vi "methane_reactor_setup.vi"() -> (2 "spec_file":path)   [LabVIEW 2019]
uses:
  lib/libSimulationControl/libSimulationControl.lvlib
  lib/libCheckpointUpdate/libCheckpointUpdate.lvlib
panel:
  # "*******************************************************************\nBiogas Plant Control\n\nAuthor: Paul Zügel\nGCSC-Frankfurt am Main 2020\n\n*******************************************************************"
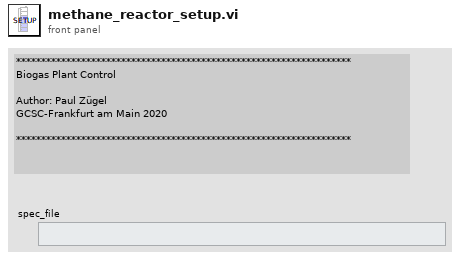
[diagram p1: front panel]
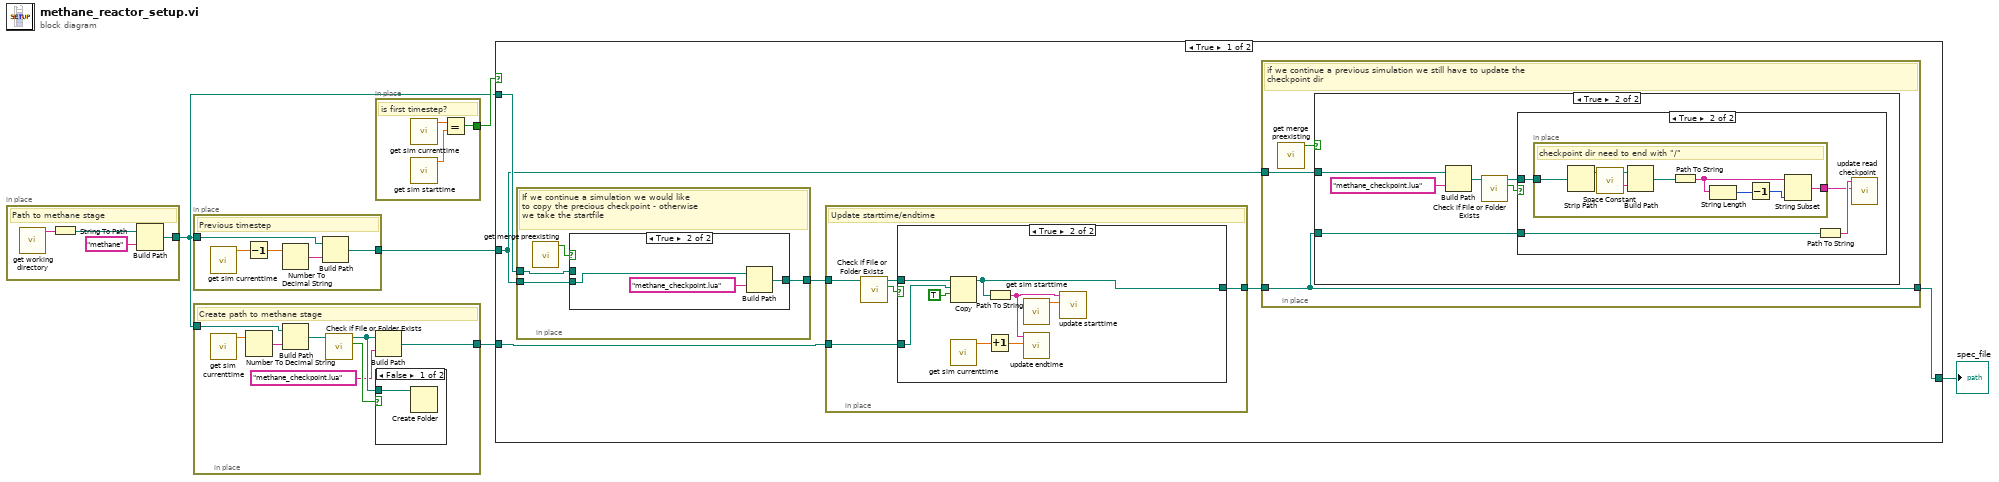
[diagram p0: block diagram]
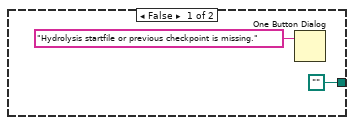
[diagram p3: hidden frame]
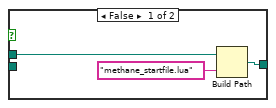
[diagram p4: hidden frame]
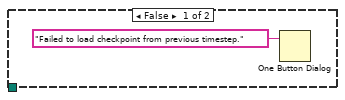
[diagram p6: hidden frame]
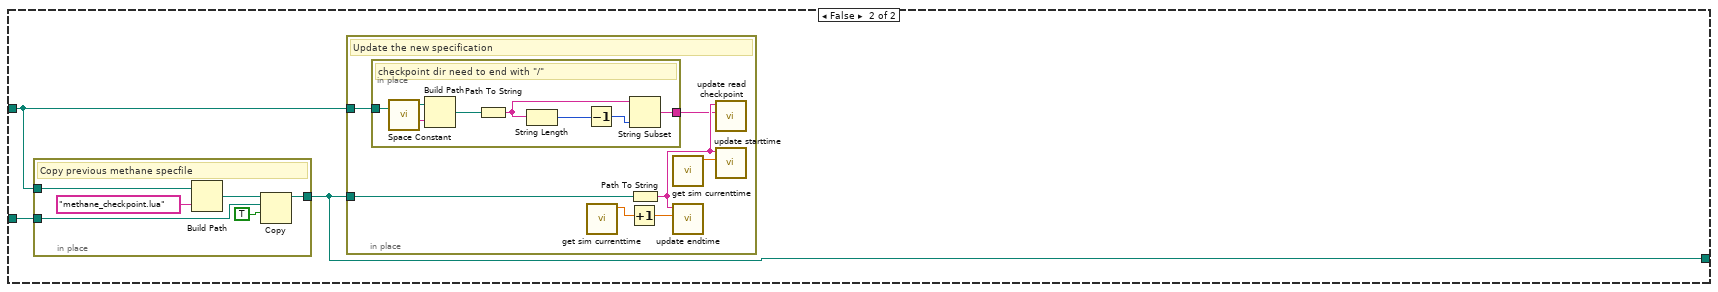
[diagram p7: hidden frame]
diagram:
  n1 = in-place {
    in-place-border: [w8] -> w1
    # "Path to methane stage"
    n2 = call "get working directory.vi"() -> ("function return"=w9:string)  [unwired: 10 in, 1 out]
    n3 = String To Path(string=w9) -> (path=w6:path)
    n4 = Build Path(base path=w6, name or relative path="methane" ("string")) -> (appended path=w8:path)
  }
  n5 = in-place {
    in-place-border: w1 -> [w13]
    in-place-border: [w11] -> w2
    # "Previous timestep"
    n6 = call "get sim currenttime.vi"() -> ("current_time"=w10:dbl)  [unwired: 10 in, 1 out]
    n7 = Decrement(x=w10) -> (x-1=w14:dbl)
    n8 = Number To Decimal String(number=w14) -> (decimal integer string=w12:string)  [unwired: 1 in]
    n9 = Build Path(base path=w13, name or relative path=w12) -> (appended path=w11:path)
  }
  n10 = in-place {
    in-place-border: [w17] -> w3
    in-place-border: w1 -> [w15]
    # "Create path to methane stage"
    n11 = call "get sim currenttime.vi"() -> ("current_time"=w16:dbl)  [unwired: 10 in, 1 out]
    n12 = Number To Decimal String(number=w16) -> (decimal integer string=w21:string)  [unwired: 1 in]
    n13 = Build Path(base path=w15, name or relative path=w21) -> (appended path=w20:path)
    n14 = call <vilib>:"Check if File or Folder Exists.vi"("path"=w20) -> ("file or folder exists?"=w22:bool, "dup path"=w19:path)  [unwired: 8 in, 1 out]
    n15 = Build Path(base path=w19, name or relative path="methane_checkpoint.lua" ("string")) -> (appended path=w17:path)
    n16 = case shown="False" w22 {
      tunnel: w19 -> [w23 _]
      frame False {
        n17 = Create Folder(path (use dialog)=w23) -> ()  [unwired: 2 in, 3 out]
      }
      frame True {
      }
    }
  }
  n18 = in-place {
    in-place-border: [w26] -> w5
    # "is first timestep?"
    n19 = call "get sim currenttime.vi"() -> ("current_time"=w24:dbl)  [unwired: 10 in, 1 out]
    n20 = call "get sim starttime.vi"() -> ("sim_starttime"=w25:dbl)  [unwired: 10 in, 1 out]
    n21 = Equal?(x=w24, y=w25) -> (x = y?=w26:bool)
  }
  n22 = case shown="True" w5 {
    tunnel: [w32 w81] -> w4
    tunnel: w3 -> [w28 w82]
    tunnel: w2 -> [w30 w80]
    tunnel: w1 -> [w31 _]
    frame True {
      n23 = in-place {
        in-place-border: [w51] -> w29
        in-place-border: w31 -> [w49]
        in-place-border: w30 -> [w48]
        # "If we continue a simulation we would like\nto copy the precious checkpoint - otherwise\nwe take the startfile"
        n24 = call "get merge preexisting.vi"() -> ("function return"=w50:bool)  [unwired: 10 in, 1 out]
        n25 = case shown="True" w50 {
          tunnel: [w53 w56] -> w51
          tunnel: w49 -> [w52 _]
          tunnel: w48 -> [_ w55]
          frame False {
            # "Copy base specification and update starttime/endtime"
            n26 = Build Path(base path=w52, name or relative path="methane_startfile.lua") -> (appended path=w53:path)
          }
          frame True {
            # "Copy previous hydrolysis spec file"
            n27 = Build Path(base path=w55, name or relative path="methane_checkpoint.lua" ("string")) -> (appended path=w56:path)
          }
        }
      }
      n28 = in-place {
        in-place-border: w29 -> [w35]
        in-place-border: w28 -> [w34]
        in-place-border: [w33] -> w27
        # "Update starttime/endtime"
        n29 = call <vilib>:"Check if File or Folder Exists.vi"("path"=w35) -> ("file or folder exists?"=w36:bool, "dup path"=w37:path)  [unwired: 8 in, 1 out]
        n30 = case shown="True" w36 {
          tunnel: [path "" w47] -> w33
          tunnel: w37 -> [_ w44]
          tunnel: w34 -> [_ w43]
          frame False {
            n31 = One Button Dialog(message="Hydrolysis startfile or previous checkpoint is missing.") -> ()  [unwired: 1 in, 1 out]
          }
          frame True {
            # "Update starttime/endtime"
            n32 = Copy(9:TRUE ("overwrite (F)"), 10:w43, 11:w44) -> (3:w47:path)  [unwired: 2 in, 2 out]
            n33 = call "get sim currenttime.vi"() -> ("current_time"=w42:dbl)  [unwired: 10 in, 1 out]
            n34 = Increment(x=w42) -> (x+1=w41:dbl)
            n35 = Path To String(path=w47) -> (string=w45:string)
            n36 = call "get sim starttime.vi"() -> ("sim_starttime"=w40:dbl)  [unwired: 10 in, 1 out]
            n37 = call "update endtime.vi"("endtime"=w41, "spec_dir"=w45) -> ()  [unwired: 9 in, 1 out]
            n38 = call "update starttime.vi"("starttime"=w40, "spec_dir"=w45) -> ()  [unwired: 9 in, 1 out]
          }
        }
      }
      n39 = in-place {
        in-place-border: w27 -> [w58]
        in-place-border: [w58] -> w32
        in-place-border: w30 -> [w59]
        # "if we continue a previous simulation we still have to update the \ncheckpoint dir"
        n40 = call "get merge preexisting.vi"() -> ("function return"=w60:bool)  [unwired: 10 in, 1 out]
        n41 = case shown="True" w60 {
          tunnel: w59 -> [_ w65]
          tunnel: w58 -> [_ w61]
          frame False {
          }
          frame True {
            n42 = Build Path(base path=w65, name or relative path="methane_checkpoint.lua" ("string")) -> (appended path=w64:path)
            n43 = call <vilib>:"Check if File or Folder Exists.vi"("path"=w64) -> ("file or folder exists?"=w62:bool, "dup path"=w63:path)  [unwired: 8 in, 1 out]
            n44 = case shown="True" w62 {
              tunnel: w63 -> [_ w69]
              tunnel: w61 -> [_ w70]
              frame False {
                n45 = One Button Dialog(message="Failed to load checkpoint from previous timestep.") -> ()  [unwired: 1 in, 1 out]
              }
              frame True {
                n46 = in-place {
                  in-place-border: w69 -> [w79]
                  in-place-border: [w72] -> w68
                  # "checkpoint dir need to end with \"/\""
                  n47 = Strip Path(path=w79) -> (stripped path=w73:path)  [unwired: 1 out]
                  n48 = call <vilib>:"Space Constant.vi"() -> ("String"=w74:string)
                  n49 = Build Path(base path=w73, name or relative path=w74) -> (appended path=w77:path)
                  n50 = Path To String(path=w77) -> (string=w78:string)
                  n51 = String Length(string=w78) -> (length=w76:i32)
                  n52 = Decrement(x=w76) -> (x-1=w75:i32)
                  n53 = String Subset(string=w78, length (rest)=w75) -> (substring=w72:string)  [unwired: 1 in]
                }
                n54 = Path To String(path=w70) -> (string=w71:string)
                n55 = call "update read checkpoint.vi"("checkpoint_dir"=w68, "spec_dir"=w71) -> ()  [unwired: 9 in, 1 out]
              }
            }
          }
        }
      }
    }
    frame False {
      n56 = in-place {
        in-place-border: w82 -> [w87]
        in-place-border: [w84] -> w81
        in-place-border: w80 -> [w83]
        # "Copy previous methane specfile"
        n57 = Build Path(base path=w83, name or relative path="methane_checkpoint.lua" ("string")) -> (appended path=w86:path)
        n58 = Copy(9:TRUE ("overwrite (F)"), 10:w87, 11:w86) -> (3:w84:path)  [unwired: 2 in, 2 out]
      }
      n59 = in-place {
        in-place-border: w81 -> [w95]
        in-place-border: w80 -> [w89]
        # "Update the new specification"
        n60 = in-place {
          in-place-border: [w97] -> w90
          in-place-border: w89 -> [w96]
          # "checkpoint dir need to end with \"/\""
          n61 = call <vilib>:"Space Constant.vi"() -> ("String"=w98:string)
          n62 = Build Path(base path=w96, name or relative path=w98) -> (appended path=w101:path)
          n63 = Path To String(path=w101) -> (string=w102:string)
          n64 = String Length(string=w102) -> (length=w100:i32)
          n65 = Decrement(x=w100) -> (x-1=w99:i32)
          n66 = String Subset(string=w102, length (rest)=w99) -> (substring=w97:string)  [unwired: 1 in]
        }
        n67 = call "get sim currenttime.vi"() -> ("current_time"=w92:dbl)  [unwired: 10 in, 1 out]
        n68 = Increment(x=w92) -> (x+1=w91:dbl)
        n69 = Path To String(path=w95) -> (string=w94:string)
        n70 = call "get sim currenttime.vi"() -> ("current_time"=w93:dbl)  [unwired: 10 in, 1 out]
        n71 = call "update endtime.vi"("endtime"=w91, "spec_dir"=w94) -> ()  [unwired: 9 in, 1 out]
        n72 = call "update read checkpoint.vi"("checkpoint_dir"=w90, "spec_dir"=w94) -> ()  [unwired: 9 in, 1 out]
        n73 = call "update starttime.vi"("starttime"=w93, "spec_dir"=w94) -> ()  [unwired: 9 in, 1 out]
      }
    }
  }
  "spec_file" <- w4
